vi "group Sync Write Change Param.vi"(6 "data_pos":u16, 7 "data_length":u16, 8 "error in (no error)":errorcluster, 9 "data":u32, 10 "id":u8, 11 "group_num":i32) -> (0 "error out":errorcluster, 3 "function return":u8)   [LabVIEW 2018, in "labview.lvlib"]
doc: "WINDECLSPEC uint8_t groupSyncWriteChangeParam (int group_num, uint8_t id, uint32_t data, uint16_t data_length, uint16_t data_pos);"
uses:
  labview.lvlib
  dxl_x86_c.dll
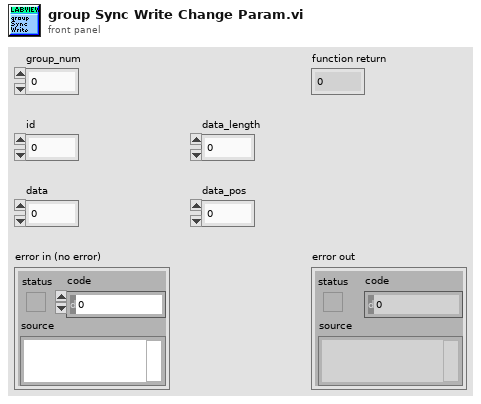
[diagram p1: front panel]
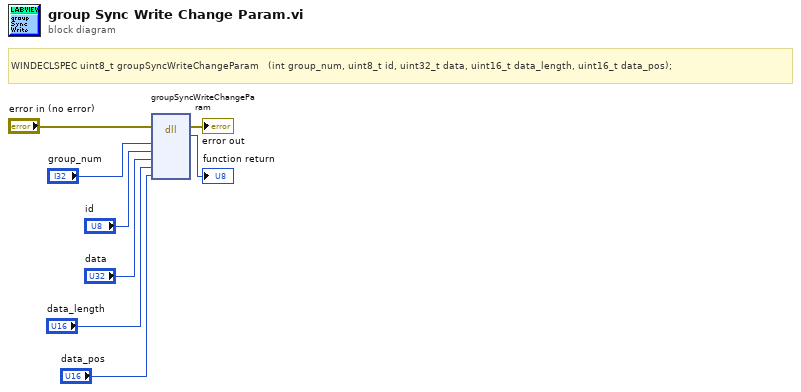
[diagram p0: block diagram]
diagram:
  # "WINDECLSPEC uint8_t groupSyncWriteChangeParam   (int group_num, uint8_t id, uint32_t data, uint16_t data_length, uint16_t data_pos);"
  n1 = dll-call lib="C:/Users/joaos/OneDrive/Documents/[PhD]/Project Omnidirectional Vehicle/Vanes/LabView_code/joaoandthethreestands/DynamixelSDK-3.7.31/labview/new_compilation/dxl_x86_c.*" fn="groupSyncWriteChangeParam"(error in="error in (no error)", "group_num"="group_num", "id"="id", "data"="data", "data_length"="data_length", "data_pos"="data_pos") -> (error out=→"error out":errorcluster, →"function return":u8)  [unwired: 7 in, 1 out]
